vi "IsSearchGoalNode.vi"(8 "error in (no error)":errorcluster, 10 "PossibleGoalNode in":refnum<data-value>, 11 "SudukuBoard in":refnum<class "SudokuBoard.lvclass">) -> (0 "error out":errorcluster, 1 "IsGoal":bool, 2 "PossibleGoalNode out":refnum<data-value>, 3 "SudukuBoard out":refnum<class "SudokuBoard.lvclass">)   [LabVIEW 2014, in "SudokuBoard.lvclass"]
uses:
  <userlib>/AdvancedDataStructures/ClassBased/Applications/SudukuSolver/SudukuBoard/SudokuBoard.lvclass
  <userlib>/AdvancedDataStructures/ClassBased/GraphNode/GraphNode.lvclass
  <userlib>/AdvancedDataStructures/ClassBased/Applications/SudukuSolver/SudukuState/SudokuState.lvclass
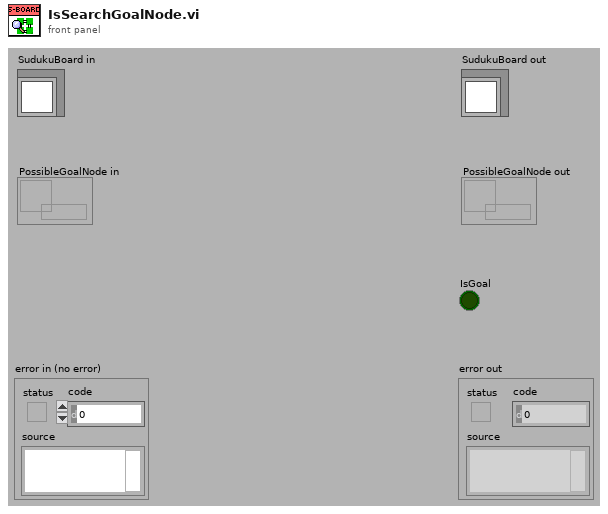
[diagram p1: front panel]
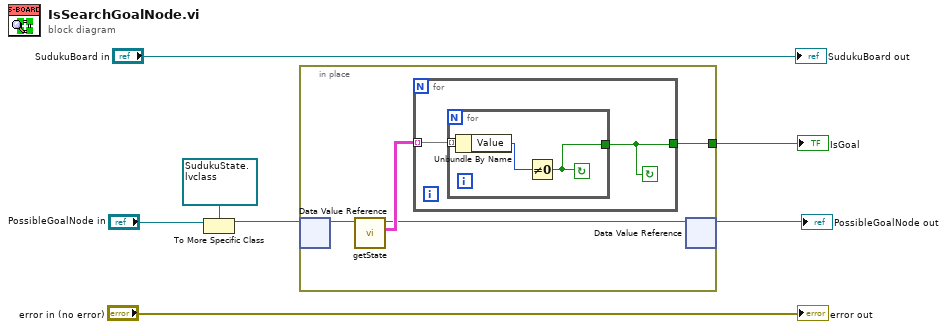
[diagram p0: block diagram]
diagram:
  n1 = To More Specific Class(target class=refnum<data-value> refnum ("data value reference"), reference="PossibleGoalNode in") -> (specific class reference=w7:refnum<data-value>)  [unwired: 1 in, 1 out]
  n2 = in-place {
    in-place-border: [w9] -> w3
    n3 = in-place-dvr #1(w7) -> (w11:refnum<class "SudokuState.lvclass">)  [unwired: 1 out]
    n4 = call <userlib>:"getState.vi"("SudukuState in"=w11) -> ("State"=w10:cluster{"Value":i32, "Options":i32[]}[][], "SudukuState out"=w8:refnum<class "SudokuState.lvclass">)  [unwired: 8 in, 1 out]
    n5 = for {
      tunnel: w10 -> [w13] mode=indexing
      tunnel: [w12] -> w9
      stop <- w12 continue-if-true
      n6 = for {
        tunnel: w13 -> [w16] mode=indexing
        tunnel: [w14] -> w12
        stop <- w14 continue-if-true
        n7 = Unbundle By Name(w16) -> ("Value"=w15:i32)
        n8 = Not Equal To 0?(x=w15) -> (x != 0?=w14:bool)
      }
    }
    n9 = in-place-dvr #1(w8) -> (→"PossibleGoalNode out":refnum<data-value>)  [unwired: 1 out]
  }
  "IsGoal" <- w3
  "error out" <- "error in (no error)"
  "SudukuBoard out" <- "SudukuBoard in"
